vi "Init.vi"(7 "Is Target?":bool, 8 "error in":errorcluster, 9 "Instr CFGs":string[](array[string]), 10 "<JSON> Virt Instr CFG":string, 11 "MSS in":refnum<class "MSS.lvclass">) -> (0 "error out":errorcluster, 1 "Target Virt Instrs":T1(array[cluster]), 2 "Target Instr CFGs":string[](array[string]), 3 "MSS out":refnum<class "MSS.lvclass">)   [LabVIEW 2024, in "HAL.lvlib" / "MSS.lvclass"]
uses:
  MSS.lvclass
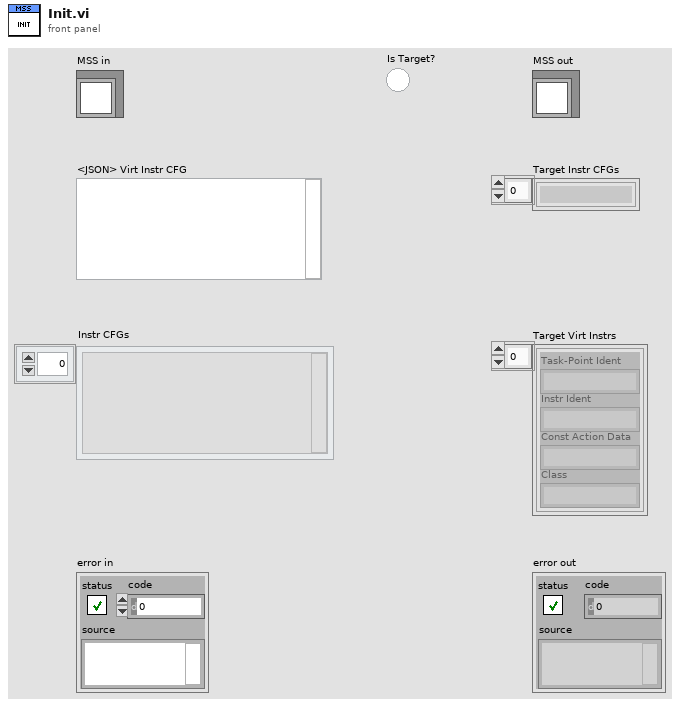
[diagram p1: front panel]
types:
  T1 = cluster{"Task-Point Ident":string, "Instr Ident":string, "Const Action Data":string, "Class":string}[]
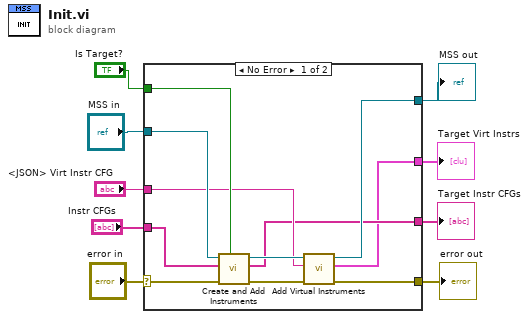
[diagram p0: block diagram]
diagram:
  n1 = case shown="No Error" "error in" {
    selector: "error in" -> [w19 w22]
    tunnel: [w18 w22] -> w8
    tunnel: [w16 w21] -> w6
    tunnel: "MSS in" -> [w17 w21]
    tunnel: "Is Target?" -> [w20 _]
    tunnel: "Instr CFGs" -> [w15 _]
    tunnel: "<JSON> Virt Instr CFG" -> [w12 _]
    tunnel: [w11 _] -> w1
    tunnel: [w10 _] -> w2
    frame No Error {
      n2 = call "Create and Add Instruments.vi"("Is Target?"=w20, "Error In"=w19, "Instr CFGs"=w15, "MSS in"=w17) -> ("Error Out"=w13:errorcluster, "Target Instr CFGs"=w11:string[], "MSS out"=w14:refnum<class "MSS.lvclass">)  [unwired: 5 in]
      n3 = call "Add Virtual Instruments.vi"("error in"=w13, "<JSON> CFG"=w12, "MSS in"=w14) -> ("error out"=w18:errorcluster, "Target Virt Instrs"=w10:T1, "MSS out"=w16:refnum<class "MSS.lvclass">)  [unwired: 6 in]
    }
    frame Error {
    }
  }
  "error out" <- w8
  "MSS out" <- w6
  "Target Virt Instrs" <- w2
  "Target Instr CFGs" <- w1
